vi "bulk_read.vi"() -> ()   [LabVIEW 2015]
uses:
  dxl_x86_c.lvlib/dxl_x86_c.lvlib
panel:
  in  "LEN_MX_\nMOVING":u16=1
  in  "ADDR_MX_\nMOVING":u16=46
  out "value : MX (LED)\nis moving 2":bool
  out "group_num":i32
  in  "LEN_MX_\nPRESENT_POSITION":u16=2
  in  "dynamixe2_id":u8=2
  in  "device_name":string="COM8"
  in  "ADDR_MX_\nPRESENT_POSITION":u16=36
  in  "ADDR_MX_\nGOAL_POSITION":u16=30
  in  "ADDR_MX_\nTORQUE_ENABLE":u16=24
  out "protocol_version":dbl=1.0
  out "value : MX (knob)\npresent position 1":u32(knob)=1962
  in  "terminate":bool
  out "port_num":i32
  in  "value : MX (dial)\ngoal position":u16(knob)=1963
  in  "dynamixel1_id":u8=1
  in  "baud_rate":i32=1000000
  # "bulk_read.vi\n\nCreated on: 2016. 6. 13\nAuthor: Leon Ryu Woon Jung\n\n*********     Bulk Read Example      *********\n\n\nAvailable Dynamixel model on this example : MX or X series set to Protocol 1.0\nThis example is designed for using two Dynamixel MX-28, and an USB2DYNAMIXEL.\nTo use another Dynamixel model, such as X series, see their details in E-Manual(support.robotis.com) and edit below variables yourself.\nBe sure that Dynamixel MX properties are already set as %% ID : 1 / Baudnum : 1 (Baudrate : 1000000)\n\n1. Run example by click above \"Run\" button (below \"Edit\" menu).\n2. Drag \"dial\" then you may see the Dynamixel and \"knob\"s rotating\n3. To finish the example, press \"terminate\" button."
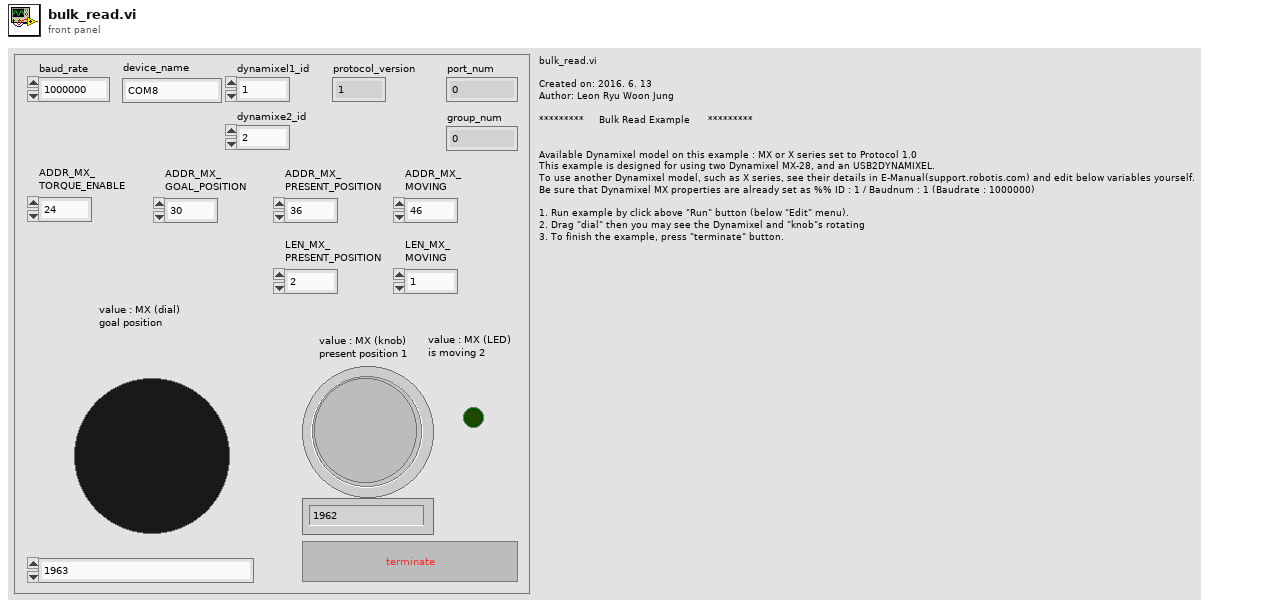
[diagram p1: front panel]
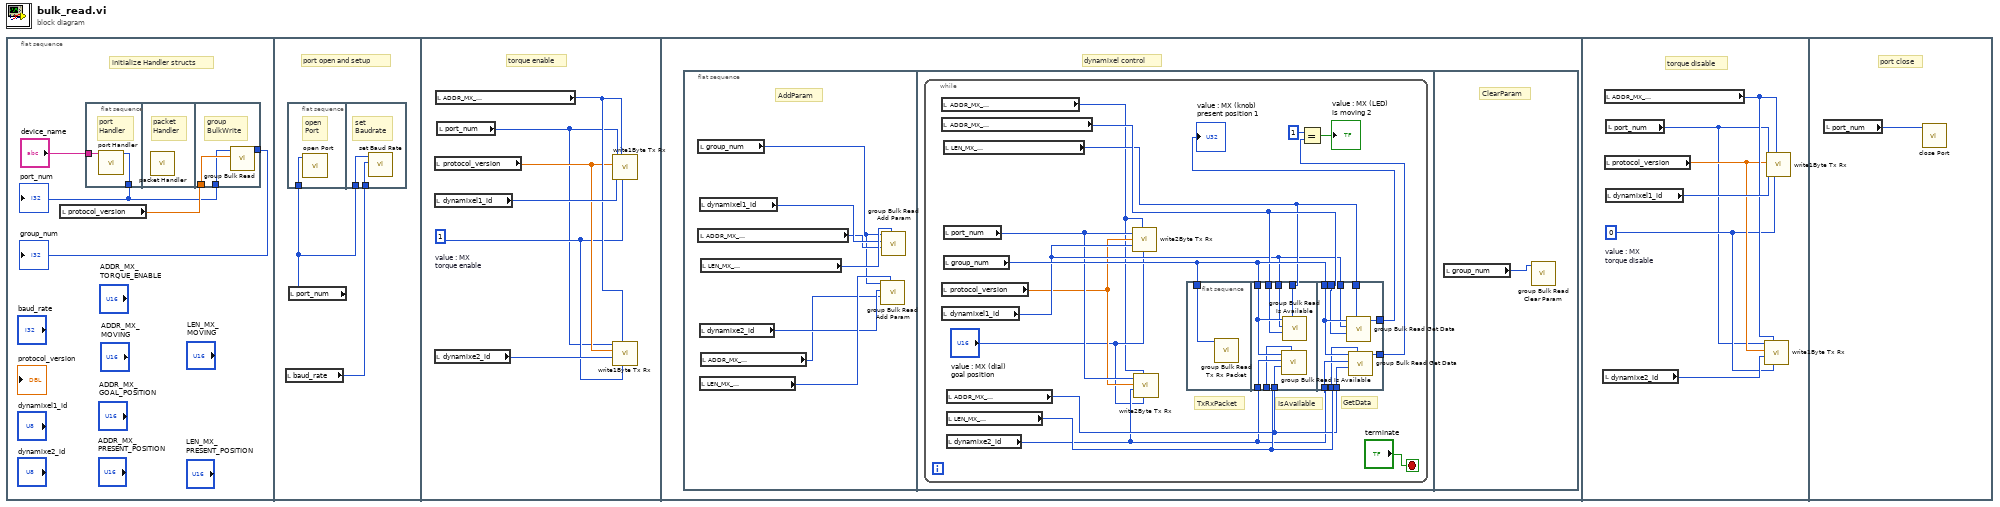
[diagram p0: block diagram]
diagram:
  n1 = flat-sequence {
    frame #0 {
      # "initialize Handler structs"
      n2 = local read "protocol_version"() -> (w3:dbl)
      n3 = flat-sequence {
        tunnel: "device_name" -> [w6]
        tunnel: [w5] -> w2
        tunnel: w3 -> [w9]
        tunnel: w2 -> [w8]
        tunnel: [w7] -> w1
        frame #0 {
          # "port\nHandler"
          n4 = call "port Handler.vi"("port_name"=w6) -> ("function return"=w5:i32)  [unwired: 10 in]
        }
        frame #1 {
          # "packet\nHandler"
          n5 = call "packet Handler.vi"() -> ()  [unwired: 12 in]
        }
        frame #2 {
          # "group\nBulkWrite"
          n6 = call "group Bulk Read.vi"("protocol_version"=w9, "port_num"=w8) -> ("function return"=w7:i32)  [unwired: 9 in]
        }
      }
      "port_num" <- w2
      "group_num" <- w1
    }
    frame #1 {
      # "port open and setup"
      n7 = local read "baud_rate"() -> (w10:i32)
      n8 = flat-sequence {
        tunnel: w11 -> [w12]
        tunnel: w11 -> [w14]
        tunnel: w10 -> [w13]
        frame #0 {
          # "open\nPort"
          n9 = call "open Port.vi"("port_num"=w12) -> ()  [unwired: 10 in, 1 out]
        }
        frame #1 {
          # "set\nBaudrate"
          n10 = call "set Baud Rate.vi"("baudrate"=w13, "port_num"=w14) -> ()  [unwired: 9 in, 1 out]
        }
      }
      n11 = local read "port_num"() -> (w11:i32)
    }
    frame #2 {
      w16 = 1  # value : MX torque enable
      # "torque enable"
      n12 = local read "protocol_version"() -> (w18:dbl)
      n13 = local read "dynamixel1_id"() -> (w20:u8)
      n14 = local read "dynamixe2_id"() -> (w17:u8)
      n15 = local read "ADDR_MX_\nTORQUE_ENABLE"() -> (w19:u16)
      n16 = local read "port_num"() -> (w15:i32)
      n17 = call "write1Byte Tx Rx.vi"("data"=w16, "address"=w19, "id"=w20, "protocol_version"=w18, "port_num"=w15) -> ()  [unwired: 7 in]
      n18 = call "write1Byte Tx Rx.vi"("data"=w16, "address"=w19, "id"=w17, "protocol_version"=w18, "port_num"=w15) -> ()  [unwired: 7 in]
    }
    frame #3 {
      # "dynamixel control"
      n19 = flat-sequence {
        frame #0 {
          # "AddParam"
          n20 = local read "group_num"() -> (w23:i32)
          n21 = local read "ADDR_MX_\nPRESENT_POSITION"() -> (w25:u16)
          n22 = local read "dynamixel1_id"() -> (w26:u8)
          n23 = local read "dynamixe2_id"() -> (w22:u8)
          n24 = local read "LEN_MX_\nMOVING"() -> (w24:u16)
          n25 = local read "LEN_MX_\nPRESENT_POSITION"() -> (w27:u16)
          n26 = local read "ADDR_MX_\nMOVING"() -> (w21:u16)
          n27 = call "group Bulk Read Add Param.vi"("data_length"=w24, "start_address"=w21, "id"=w22, "group_num"=w23) -> ()  [unwired: 7 in, 1 out]
          n28 = call "group Bulk Read Add Param.vi"("data_length"=w27, "start_address"=w25, "id"=w26, "group_num"=w23) -> ()  [unwired: 7 in, 1 out]
        }
        frame #1 {
          n29 = while {
            stop <- "terminate" stop-if-true
            # "TxRxPacket"
            # "IsAvailable"
            # "GetData"
            n30 = local read "ADDR_MX_\nGOAL_POSITION"() -> (w28:u16)
            n31 = local read "ADDR_MX_\nPRESENT_POSITION"() -> (w41:u16)
            n32 = local read "protocol_version"() -> (w31:dbl)
            n33 = local read "dynamixel1_id"() -> (w33:u8)
            n34 = local read "LEN_MX_\nPRESENT_POSITION"() -> (w34:u16)
            n35 = local read "port_num"() -> (w32:i32)
            n36 = local read "group_num"() -> (w42:i32)
            n37 = local read "ADDR_MX_\nMOVING"() -> (w35:u16)
            n38 = local read "LEN_MX_\nMOVING"() -> (w40:u16)
            n39 = local read "dynamixe2_id"() -> (w30:u8)
            n40 = call "write2Byte Tx Rx.vi"("data"="value : MX (dial)\ngoal position", "address"=w28, "id"=w33, "protocol_version"=w31, "port_num"=w32) -> ()  [unwired: 7 in]
            n41 = call "write2Byte Tx Rx.vi"("data"="value : MX (dial)\ngoal position", "address"=w28, "id"=w30, "protocol_version"=w31, "port_num"=w32) -> ()  [unwired: 7 in]
            n42 = flat-sequence {
              tunnel: w42 -> [w44]
              tunnel: w42 -> [w51]
              tunnel: w30 -> [w50]
              tunnel: w41 -> [w49]
              tunnel: w40 -> [w48]
              tunnel: w35 -> [w47]
              tunnel: w34 -> [w46]
              tunnel: w33 -> [w45]
              tunnel: w42 -> [w60]
              tunnel: w30 -> [w59]
              tunnel: w41 -> [w58]
              tunnel: w40 -> [w55]
              tunnel: [w57] -> w37
              tunnel: [w56] -> w36
              tunnel: w35 -> [w54]
              tunnel: w34 -> [w53]
              tunnel: w33 -> [w52]
              frame #0 {
                n43 = call "group Bulk Read Tx Rx Packet.vi"("group_num"=w44) -> ()  [unwired: 11 in]
              }
              frame #1 {
                n44 = call "group Bulk Read Is Available.vi"("data_length"=w48, "address"=w47, "id"=w50, "group_num"=w51) -> ()  [unwired: 7 in, 1 out]
                n45 = call "group Bulk Read Is Available.vi"("data_length"=w46, "address"=w49, "id"=w45, "group_num"=w51) -> ()  [unwired: 7 in, 1 out]
              }
              frame #2 {
                n46 = call "group Bulk Read Get Data.vi"("data_length"=w53, "address"=w58, "id"=w52, "group_num"=w60) -> ("function return"=w56:u32)  [unwired: 7 in]
                n47 = call "group Bulk Read Get Data.vi"("data_length"=w55, "address"=w54, "id"=w59, "group_num"=w60) -> ("function return"=w57:u32)  [unwired: 7 in]
              }
            }
            n48 = Equal?(x=1, y=w37) -> (x = y?=→"value : MX (LED)\nis moving 2":bool)
            "value : MX (knob)\npresent position 1" <- w36
          }
        }
        frame #2 {
          # "ClearParam"
          n49 = local read "group_num"() -> (w61:i32)
          n50 = call "group Bulk Read Clear Param.vi"("group_num"=w61) -> ()  [unwired: 11 in]
        }
      }
    }
    frame #4 {
      w63 = 0  # value : MX torque disable
      # "torque disable"
      n51 = local read "dynamixe2_id"() -> (w64:u8)
      n52 = local read "ADDR_MX_\nTORQUE_ENABLE"() -> (w66:u16)
      n53 = local read "protocol_version"() -> (w65:dbl)
      n54 = local read "dynamixel1_id"() -> (w67:u8)
      n55 = local read "port_num"() -> (w62:i32)
      n56 = call "write1Byte Tx Rx.vi"("data"=w63, "address"=w66, "id"=w64, "protocol_version"=w65, "port_num"=w62) -> ()  [unwired: 7 in]
      n57 = call "write1Byte Tx Rx.vi"("data"=w63, "address"=w66, "id"=w67, "protocol_version"=w65, "port_num"=w62) -> ()  [unwired: 7 in]
    }
    frame #5 {
      # "port close"
      n58 = local read "port_num"() -> (w68:i32)
      n59 = call "close Port.vi"("port_num"=w68) -> ()  [unwired: 11 in]
    }
  }
